vi "countFTrunNoofLot.vi"(11 "Lotno":string) -> (3 "data":i32)   [LabVIEW 2012]
uses:
  <vilib>/addons/database/Auxilliary.llb/DB Tools Cursor Type.ctl
  Global1.vi
  <vilib>/addons/database/Connection.llb/DB Tools Open Connec (Path).vi
  <vilib>/addons/database/Connection.llb/Conn Execute.vi
  <vilib>/addons/database/Recordset.llb/Rec Fetch Integer Data (R).vi
  <vilib>/addons/database/Recordset.llb/Rec Destroy - Connection.vi
  <vilib>/addons/database/NI_Database_API.lvlib
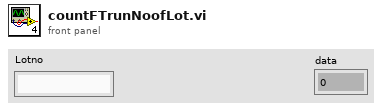
[diagram p1: front panel]
types:
  T1 = typedef "NI_Database_API.lvlib/DB Tools Cursor Type.ctl" = enum16{"forward-only", "keyset", "dynamic", "static"}
  T2 = typedef "NI_Database_API.lvlib/Conn ObjectReference.ctl" = refnum<k1>
  T3 = typedef "NI_Database_API.lvlib/Rec ObjectReference.ctl" = refnum<k1>
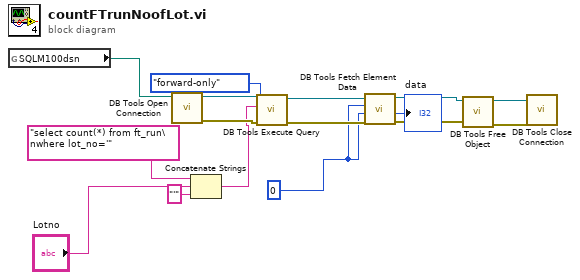
[diagram p0: block diagram]
diagram:
  w3 = 0
  n1 = global read "Global1.vi" "SQLM100dsn"() -> (w1:path)
  n2 = call-poly <vilib>:"DB Tools Open Connection.vi"("connection information"=w1) -> ("error out"=w12:errorcluster, "connection reference"=w16:T2)  [unwired: 7 in]
  n3 = Concatenate Strings("select count(*) from ft_run\nwhere lot_no='" ("string"), "Lotno", "'" ("string")) -> (w5:string)
  n4 = call-poly <vilib>:"DB Tools Execute Query.vi"("error in (no error)"=w12, "cursor type"=DB_Tools_Cursor_Type."forward-only", "SQL query"=w5, "connection reference"=w16) -> ("error out"=w11:errorcluster, "recordset reference"=w15:T3)  [unwired: 4 in]
  n5 = call-poly <vilib>:"DB Tools Fetch Element Data.vi"("error in (no error)"=w11, "type"=w3, "column index"=w3, "recordset reference"=w15) -> ("error out"=w10:errorcluster, "data"=→"data":i32, "recordset reference out"=w14:T3)  [unwired: 3 in]
  n6 = call-poly <vilib>:"DB Tools Free Object.vi"("error in (no error)"=w10, "recordset reference"=w14) -> ("error out"=w9:errorcluster, "connection reference"=w13:T2)  [unwired: 8 in]
  n7 = call <vilib>:"DB Tools Close Connection.vi"("error in (no error)"=w9, "connection reference"=w13) -> ()  [unwired: 5 in, 1 out]
